vi "Set Item Selection.vi"(8 "error in (no error)":errorcluster, 9 "Selected?":bool, 10 "Tag":string, 11 "TreeSelection in":refnum<class "TreeSelection.lvclass">) -> (0 "error out":errorcluster, 3 "TreeSelection out":refnum<class "TreeSelection.lvclass">)   [LabVIEW 2015, in "TreeSelection.lvclass"]
doc: "<b> </b> <b> </b>\n©2016 Q Software Innovations, LLC (QSI)\nwritten by Quentin Alldredge\nproduced in LabVIEW 2015\n\nsupport@qsoftwareinnovations.com\nwww.qsoftwareinnovations.com\n\nAll rights reserved.\n\nRedistribution and use in source and binary forms, with or without modification, are permitted provided that the following conditions are met:\n\n * Redistributions of source code must retain the above copyright notice, this list of conditions and the following disclaimer.\n * Redistributions in binary form must reproduce the above copyright notice, this list of conditions and the following disclaimer in the documentation and/or other materials provided with the distribution.\n * Neither the name of Q Software Innovations, LLC. nor the names of its contributors may be used to endorse or promote products derived from this software without specific prior written permission.\n\nTHIS SOFTWARE IS PROVIDED BY THE COPYRIGHT HOLDERS AND CONTRIBUTORS \"AS IS\" AND ANY EXPRESS OR IMPLIED WARRANTIES, INCLUDING, BUT NOT LIMITED TO, THE IMPLIED WARRANTIES OF MERCHANTABILITY AND FITNESS FOR A PARTICULAR PURPOSE ARE DISCLAIMED. IN NO EVENT SHALL THE COPYRIGHT OWNER OR CONTRIBUTORS BE LIABLE FOR ANY DIRECT, INDIRECT, INCIDENTAL, SPECIAL, EXEMPLARY, OR CONSEQUENTIAL DAMAGES (INCLUDING, BUT NOT LIMITED TO, PROCUREMENT OF SUBSTITUTE GOODS OR SERVICES; LOSS OF USE, DATA, OR PROFITS; OR BUSINESS INTERRUPTION) HOWEVER CAUSED AND ON ANY THEORY OF LIABILITY, WHETHER IN CONTRACT, STRICT LIABILITY, OR TORT (INCLUDING NEGLIGENCE OR OTHERWISE) ARISING IN ANY WAY OUT OF THE USE OF THIS SOFTWARE, EVEN IF ADVISED OF THE POSSIBILITY OF SUCH DAMAGE."
uses:
  TreeSelection.lvclass
  TreeControl/TreeControl.lvclass
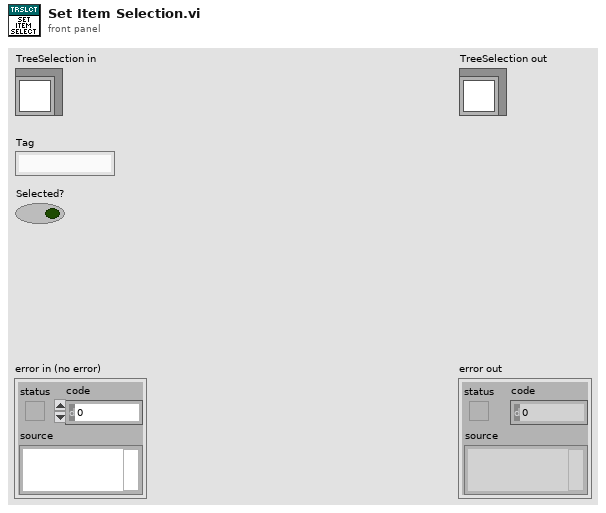
[diagram p1: front panel]
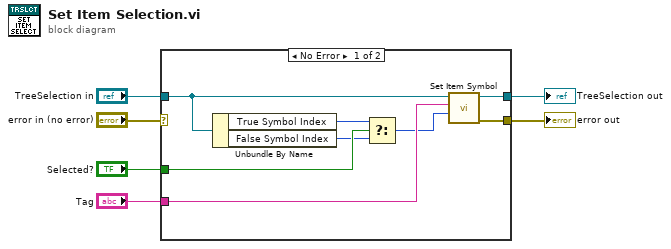
[diagram p0: block diagram]
diagram:
  n1 = case shown="No Error" "error in (no error)" {
    selector: "error in (no error)" -> [_ w16]
    tunnel: [w7 w16] -> w5
    tunnel: [w13 w15] -> w3
    tunnel: "TreeSelection in" -> [w14 w15]
    tunnel: "Tag" -> [w12 _]
    tunnel: "Selected?" -> [w11 _]
    frame No Error {
      n2 = Unbundle By Name(w14) -> ("True Symbol Index"=w10:i32, "False Symbol Index"=w9:i32)
      n3 = Select(t=w10, s=w11, f=w9) -> (s? t:f=w8:i32)
      n4 = call "Set Item Symbol.vi"("Symbol Index"=w8, "Tag"=w12, "Tree in"=w14) -> ("error out"=w7:errorcluster, "Tree (dup)"=w13:refnum<class "TreeSelection.lvclass">)  [unwired: 7 in]
    }
    frame Error {
    }
  }
  "error out" <- w5
  "TreeSelection out" <- w3
